vi "RVC Two-link serial robot.vi"() -> ()   [LabVIEW 2013]
uses:
  <vilib>/Analysis/Matrix/Datatypes/RealMatrix.ctl
  <vilib>/robotics/Kinematics/Analytical/Initialize Generic Serial Arm.vi
  <vilib>/robotics/Kinematics/Analytical/NI_Robotics_AnalyticKinematics.lvlib
  <vilib>/robotics/Kinematics/Robot/NI_Robotics_Serial Robot Arm.lvclass
  <vilib>/robotics/Kinematics/DH Kinematic Parameters.ctl
  <vilib>/robotics/Kinematics/Link/Joint Type.ctl
  <vilib>/robotics/Kinematics/Link/NI_Robotics_Link.lvclass
  <vilib>/Analysis/Matrix/NI_Matrix.lvlib
panel:
  out "forward kinematics":T1
  out "3D Picture":refnum<vi>(3d-picture)
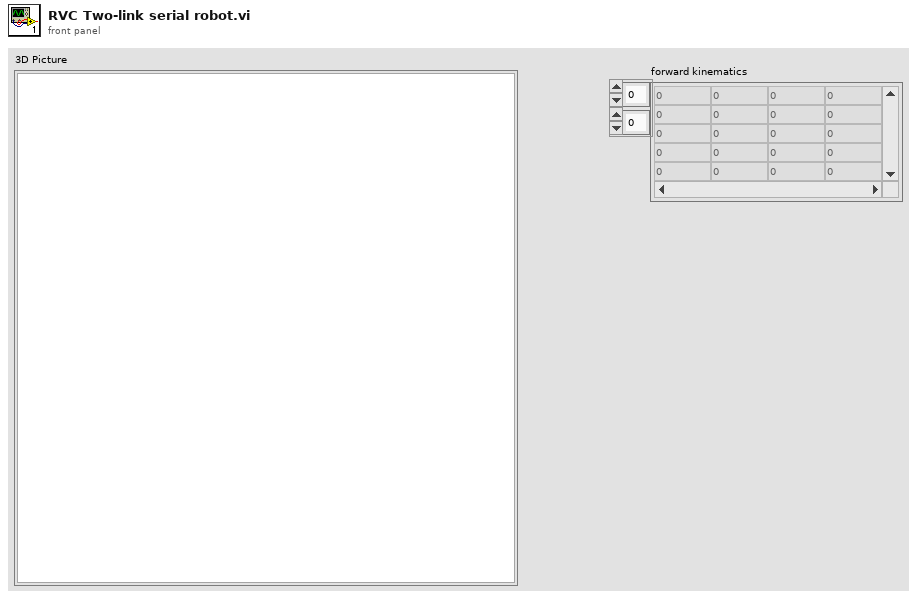
[diagram p1: front panel]
types:
  T1 = typedef "NI_Matrix.lvlib/RealMatrix.ctl" = dbl[][]
  T2 = typedef "DH Kinematic Parameters.ctl" = cluster{"twist angle":dbl, "length":dbl, "rotation angle":dbl, "offset distance":dbl, "joint type":T3, "joint coordinate offset":dbl}
  T3 = typedef "NI_Robotics_Link.lvclass/Joint Type.ctl" = enum16{"Revolute", "Prismatic"}
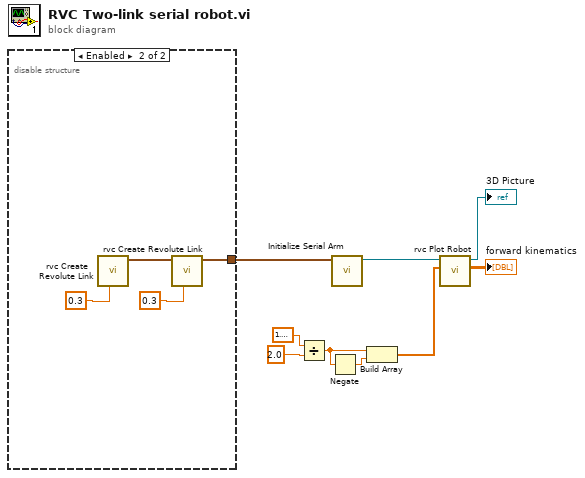
[diagram p0: block diagram]
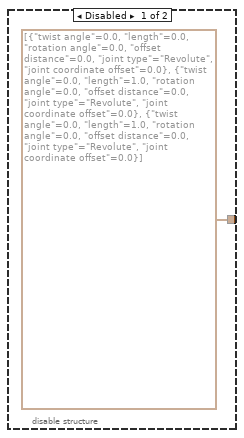
[diagram p2: hidden frame]
diagram:
  n1 = disable-structure shown="Enabled" {
    disable-tunnel: [T2[] [{"twist angle"=0.0, "length"=0.0, "rotation angle"=0.0, "offset distance"=0.0, "joint type"=enum."Revolute", "joint coordinate offset"=0.0}, {"twist angle"=0.0, "length"=1.0, "rotation angle"=0.0, "offset distance"=0.0, "joint type"=enum."Revolute", "joint coordinate offset"=0.0}, {"twist angle"=0.0, "length"=1.0, "rotation angle"=0.0, "offset distance"=0.0, "joint type"=enum."Revolute", "joint coordinate offset"=0.0}] ("kinematic parameters") w13] -> w9
    frame Disabled {
    }
    frame Enabled {
      n2 = call "rvc Create Revolute Link.vi"("length (a)"=0.3) -> ("Array"=w14:T2[])  [unwired: 10 in]
      n3 = call "rvc Create Revolute Link.vi"("length (a)"=0.3, "Array 2"=w14) -> ("Array"=w13:T2[])  [unwired: 9 in]
    }
  }
  n4 = Divide(x=1.5707963267948966, y=2.0) -> (x/y=w4:dbl)
  n5 = Negate(x=w4) -> (-x=w3:dbl)
  n6 = call-poly <vilib>:"Initialize Serial Arm.vi"("kinematic parameters"=w9) -> ("serial arm out"=w8:refnum<class "NI_Robotics_Serial Robot Arm.lvclass">)  [unwired: 9 in, 1 out]
  n7 = Build Array(w4, w3) -> (w1:dbl[])
  n8 = call "rvc Plot Robot.vi"("joint positions"=w1, "NI_Robotics_Serial Robot Arm in"=w8) -> ("forward kinematics"=→"forward kinematics":T1, "Scene Object Out"=→"3D Picture":refnum<vi>)  [unwired: 8 in]
